vi "Query First Example.vi"() -> ()   [LabVIEW 2020, in "ORM_Examples.lvlib"]
doc: "Returns the first row of the result set for the query. Note that bbPlayers and BB Players Map classes are not needed for this example."
uses:
  ORM_Examples.lvlib
  2ebe6052-648d-437f-95a6-7488cd4d4dff.vi
  2ebe6052-648d-437f-95a6-7488cd4d4dff.vi/1d2ecee2-7c09-4402-8905-d27177266061.vi
  2ebe6052-648d-437f-95a6-7488cd4d4dff.vi/bd23ee19-7bd1-410a-a455-250ae7eff562.vi
  <vilib>/Viviota/shared/ORM_ADONet.lvlibp/ADOMapper/ADOMapper.lvclass
  C:/Program Files/National Instruments/LabVIEW 2024/vi.lib/Viviota/shared/ORM.lvlibp/ORM/SqlMapper/SqlMapper.lvclass
  <vilib>/Viviota/shared/ORM_DBC_Sqlite.lvlibp/Sqlite Connect.vi
  <vilib>/Viviota/shared/ORM.lvlibp/ORM/TypeMap/ToLabVIEW_Wrap.vi
  <vilib>/Viviota/shared/ORM.lvlibp/ORM/TypeMap/TypeMap.lvclass
  <vilib>/Viviota/shared/ORM.lvlibp/ORM/DynamicParameters/DynamicParameters.lvclass
  ORM_API/ORM_API.lvlib
  <vilib>/Viviota/shared/ORM_ADONet.lvlibp
  <vilib>/Viviota/shared/ORM_DBC_Sqlite.lvlibp/DBC.lvclass
  C:/Program Files/National Instruments/LabVIEW 2024/vi.lib/Viviota/shared/ORM_ADONet.lvlibp/ADOMapper/ADOMapper.lvclass
panel:
  out "queryResult":variant
  in  "sqlQuery":string
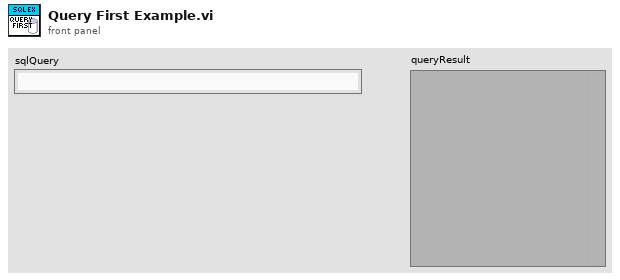
[diagram p1: front panel]
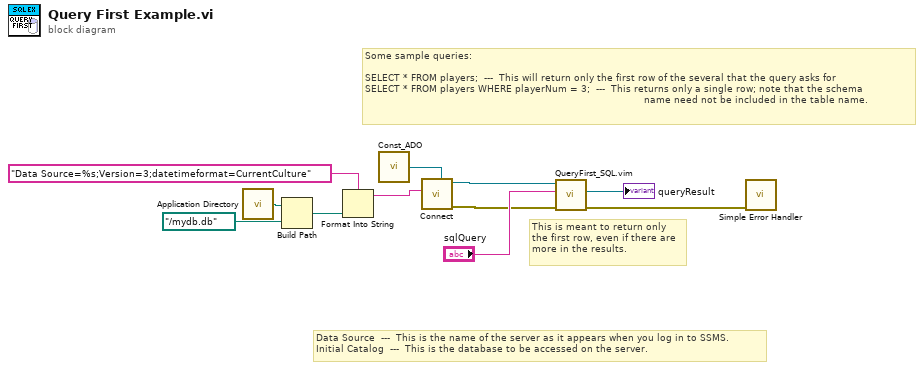
[diagram p0: block diagram]
diagram:
  # "This is meant to return only\nthe first row, even if there are\nmore in the results."
  # "Data Source  ---  This is the name of the server as it appears when you log in to SSMS.\nInitial Catalog  ---  This is the database to be accessed on the server."
  # "Some sample queries:\n\nSELECT * FROM players;  ---  This will return only the first row of the several that the query asks for\nSELECT * FROM players WHERE playerNum = 3;  ---  This returns only a single row; note that the schema\n                                                                                             name need not be included in the table name."
  n1 = call <vilib>:"Application Directory.vi"() -> ("Application Directory"=w7:path)
  n2 = Build Path(base path=w7, name or relative path=path "../mydb.db" ("file out")) -> (appended path=w8:path)
  n3 = Format Into String(format string="Data Source=%s;Version=3;datetimeformat=CurrentCulture" ("connectionStringName"), w8) -> (resulting string=w3:string)  [unwired: 2 in, 1 out]
  n4 = call <vilib>:"Const_ADO.vi"() -> ("ADOMapper"=w4:refnum<class "ADOMapper.lvclass">)
  n5 = call-poly "Connect.vi"("SqlMapper Type"=w4, "Connection String"=w3) -> ("error out"=w1:errorcluster, "SqlMapper out"=w2:refnum<class "ADOMapper.lvclass">)  [unwired: 8 in]
  n6 = call "QueryFirst_SQL.vim"("error in (no error)"=w1, "sql"="sqlQuery", "SqlMapper in"=w2) -> ("error out"=w11:errorcluster, "Value"=→"queryResult":refnum<class>)  [unwired: 6 in, 1 out]
  n7 = call <vilib>:"Simple Error Handler.vi"("error in (no error)"=w11) -> ()  [unwired: 4 in, 5 out]
